vi "microFPGA_TTL_addr_30_ctrl.vi"(0 "VISA resource name":refnum<visa-resource-name>, 1 "TTL channel":u16(ring)=3 items=["channel No 0", "channel No 1", "channel No 2", "channel No 3", "channel No 4", "channel No 5", "channel No 6"], 2 "write or read":u16(ring) items=["read", "write"], 5 "TTL mode":u16(ring) items=["LO", "HIGH"], 11 "error in (no error)":errorcluster) -> (4 "VISA out":refnum<visa-resource-name>, 6 "TTL mode read":u16(ring) items=["LO", "HIGH"], 8 "value confirm":bool, 10 "abort_wrong_input":bool, 15 "error out":errorcluster)   [LabVIEW 2018]
panel:
  out "mode read string answer":string
  out "mode read string":string
  out "mode write string":string
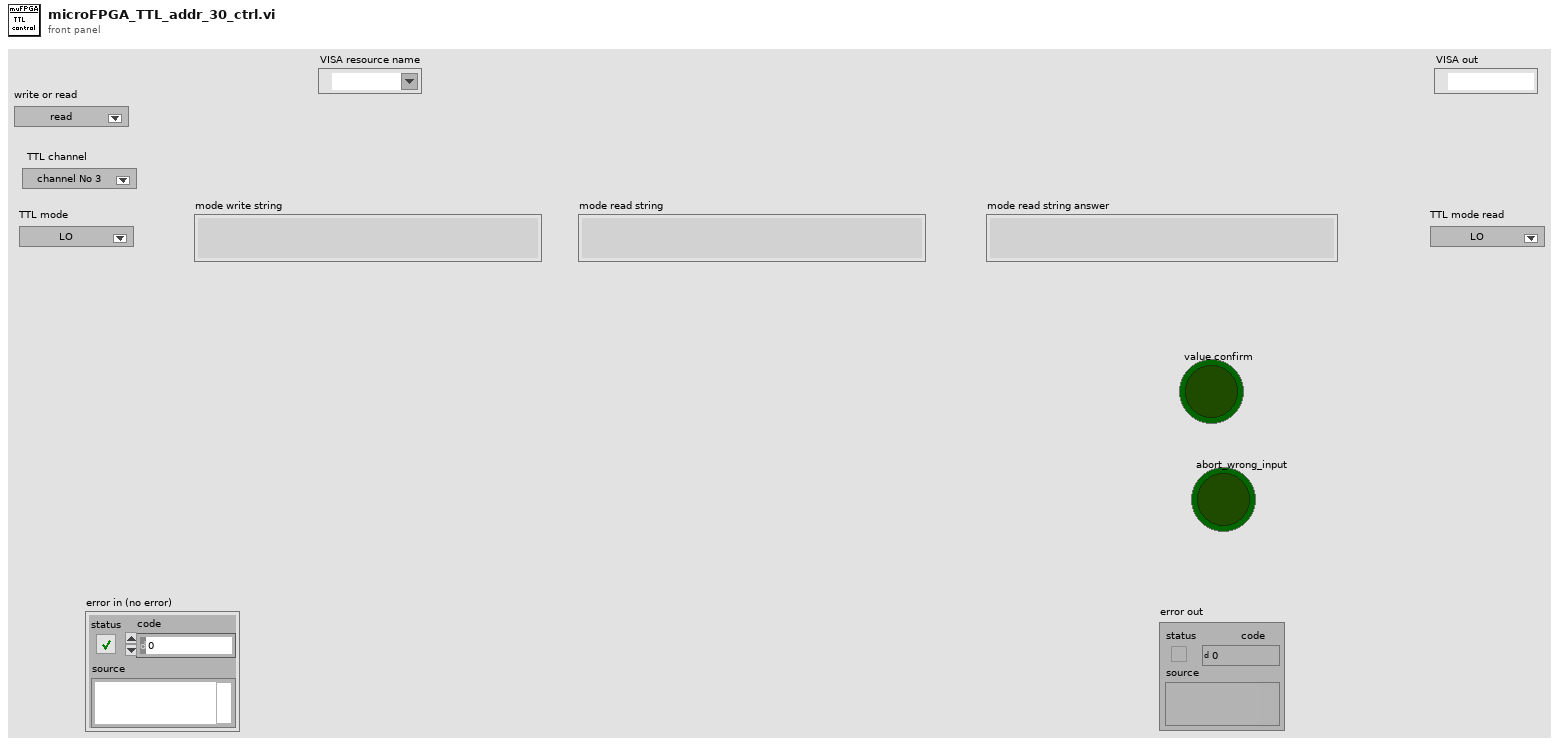
[diagram p1: front panel]
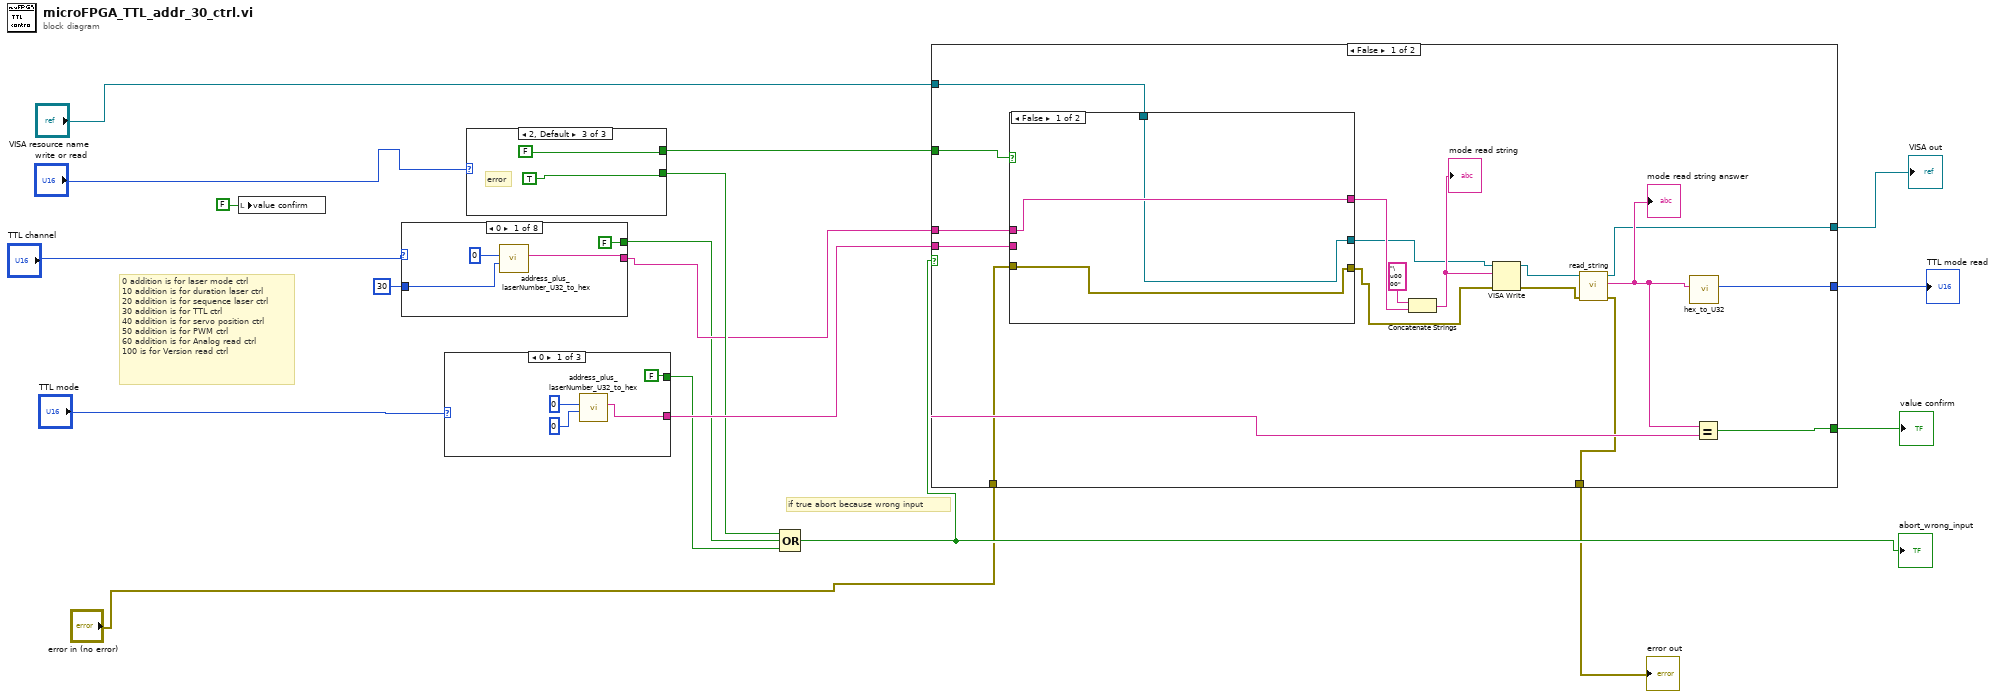
[diagram p0: block diagram]
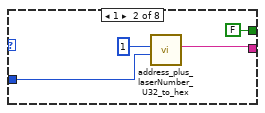
[diagram p2: hidden frame]
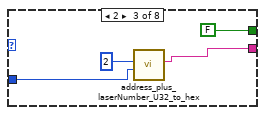
[diagram p3: hidden frame]
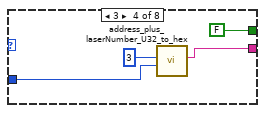
[diagram p4: hidden frame]
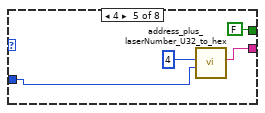
[diagram p5: hidden frame]
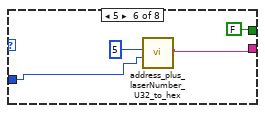
[diagram p6: hidden frame]
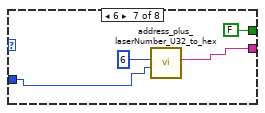
[diagram p7: hidden frame]
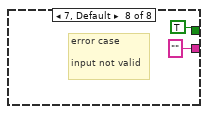
[diagram p8: hidden frame]
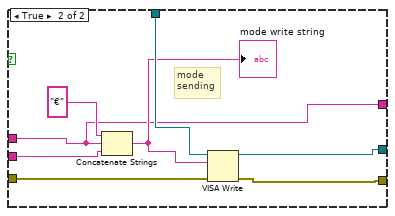
[diagram p9: hidden frame]
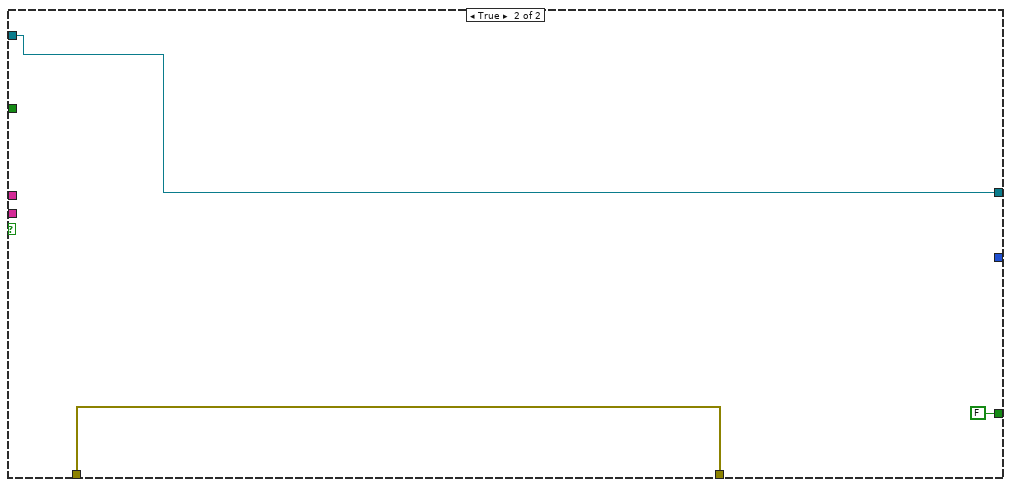
[diagram p10: hidden frame]
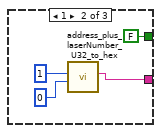
[diagram p11: hidden frame]
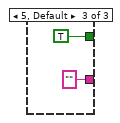
[diagram p12: hidden frame]
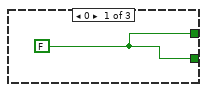
[diagram p13: hidden frame]
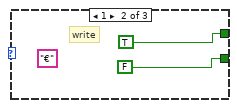
[diagram p14: hidden frame]
diagram:
  # "0 addition is for laser mode ctrl\n10 addition is for duration laser ctrl\n20 addition is for sequence laser ctrl\n30 addition is for TTL ctrl\n40 addition is for servo position ctrl\n50 addition is for PWM ctrl\n60 addition is for Analog read ctrl\n100 is for Version read ctrl"
  # "if true abort because wrong input"
  n1 = local write "value confirm"(FALSE ("value confirm")) -> ()
  n2 = case shown="0" "TTL channel" {
    tunnel: [w20 w24 w28 w32 w36 w40 w44 "" ("string 5")] -> w3
    tunnel: [FALSE FALSE FALSE FALSE FALSE FALSE FALSE TRUE] -> w2
    tunnel: u32 30 ("adress offset") -> [w19 w23 w27 w31 w35 w39 w43 _]
    frame 0 {
      n3 = call "address_plus_laserNumber_U32_to_hex.vi"("adress offset"=w19, "y 3"=u32 0) -> ("string 5"=w20:string)  [unwired: 8 in]
    }
    frame 1 {
      n4 = call "address_plus_laserNumber_U32_to_hex.vi"("adress offset"=w23, "y 3"=u32 1) -> ("string 5"=w24:string)  [unwired: 8 in]
    }
    frame 2 {
      n5 = call "address_plus_laserNumber_U32_to_hex.vi"("adress offset"=w27, "y 3"=u32 2) -> ("string 5"=w28:string)  [unwired: 8 in]
    }
    frame 3 {
      n6 = call "address_plus_laserNumber_U32_to_hex.vi"("adress offset"=w31, "y 3"=u32 3) -> ("string 5"=w32:string)  [unwired: 8 in]
    }
    frame 4 {
      n7 = call "address_plus_laserNumber_U32_to_hex.vi"("adress offset"=w35, "y 3"=u32 4) -> ("string 5"=w36:string)  [unwired: 8 in]
    }
    frame 5 {
      n8 = call "address_plus_laserNumber_U32_to_hex.vi"("adress offset"=w39, "y 3"=u32 5) -> ("string 5"=w40:string)  [unwired: 8 in]
    }
    frame 6 {
      n9 = call "address_plus_laserNumber_U32_to_hex.vi"("adress offset"=w43, "y 3"=u32 6) -> ("string 5"=w44:string)  [unwired: 8 in]
    }
    frame 7, Default {
      # "error case\n\ninput not valid"
    }
  }
  n10 = case shown="0" "TTL mode" {
    tunnel: [w49 w54 "" ("string 5")] -> w14
    tunnel: [FALSE FALSE TRUE] -> w10
    frame 0 {
      n11 = call "address_plus_laserNumber_U32_to_hex.vi"("adress offset"=u32 0, "y 3"=u32 0) -> ("string 5"=w49:string)  [unwired: 8 in]
    }
    frame 1 {
      n12 = call "address_plus_laserNumber_U32_to_hex.vi"("adress offset"=u32 0, "y 3"=u32 1) -> ("string 5"=w54:string)  [unwired: 8 in]
    }
    frame 5, Default {
    }
  }
  n13 = case shown="2, Default" "write or read" {
    tunnel: [w59 TRUE FALSE] -> w15
    tunnel: [w59 FALSE TRUE] -> w11
    frame 0 {
      w59 = FALSE
    }
    frame 1 {
      (unwired) "€" ("hex")
      # "write"
    }
    frame 2, Default {
      # "error"
    }
  }
  n14 = Compound Arithmetic op=OR(w11, w2, w10) -> (w8:bool)
  "abort_wrong_input" <- w8
  n15 = case shown="False" w8 {
    tunnel: "VISA resource name" -> [w80 w93]
    tunnel: w3 -> [w77 _]
    tunnel: w15 -> [w71 _]
    tunnel: [w70 _] -> w5
    tunnel: w14 -> [w68 _]
    tunnel: [w67 FALSE] -> w13
    tunnel: [w66 w93] -> w9
    tunnel: "error in (no error)" -> [w65 w92]
    tunnel: [w64 w92] -> w6
    frame False {
      n16 = case shown="False" w71 {
        tunnel: w77 -> [w83 w88]
        tunnel: w80 -> [w82 w90]
        tunnel: [w83 w88] -> w78
        tunnel: w68 -> [_ w87]
        tunnel: [w82 w86] -> w73
        tunnel: [w81 w85] -> w72
        tunnel: w65 -> [w81 w84]
        frame False {
        }
        frame True {
          # "mode \nsending"
          n17 = Concatenate Strings("€" ("string"), w88, w87) -> (w89:string)
          "mode write string" <- w89
          n18 = VISA Write(VISA resource name=w90, write buffer=w89, error in (no error)=w84) -> (VISA resource name out=w86:refnum<visa-resource-name>, error out=w85:errorcluster)  [unwired: 1 out]
        }
      }
      n19 = Concatenate Strings("\u0000" ("string"), w78) -> (w76:string)
      "mode read string" <- w76
      n20 = VISA Write(VISA resource name=w73, write buffer=w76, error in (no error)=w72) -> (VISA resource name out=w75:refnum<visa-resource-name>, error out=w74:errorcluster)  [unwired: 1 out]
      n21 = call "read_string.vi"("error in (no error)"=w74, "VISA resource name 2"=w75) -> ("error out"=w64:errorcluster, "read buffer"=w69:string, "VISA resource name"=w66:refnum<visa-resource-name>)  [unwired: 7 in]
      "mode read string answer" <- w69
      n22 = call "hex_to_U32.vi"("hex"=w69) -> ("U32"=w70:u32)  [unwired: 9 in]
      n23 = Equal?(x=w69, y=w68) -> (x = y?=w67:bool)
    }
    frame True {
    }
  }
  "value confirm" <- w13
  "VISA out" <- w9
  "error out" <- w6
  "TTL mode read" <- w5
